vi "FTW-JSON-SerializeElement.vi"(0 "JSON Object":refnum<class "FTW-JSON.lvclass">, 5 "Key":string, 11 "error in":errorcluster) -> (4 "JSON Object":refnum<class "FTW-JSON.lvclass">, 6 "Element as JSON String":string, 10 "Found?":bool, 15 "error out":errorcluster)   [LabVIEW 2013, in "FTW-JSON.lvclass"]
uses:
  FTW-JSON.lvclass
  FTW-JSON.lvclass/FTW-JSON.ctl
panel:
  # "Inputs"
  # "Outputs"
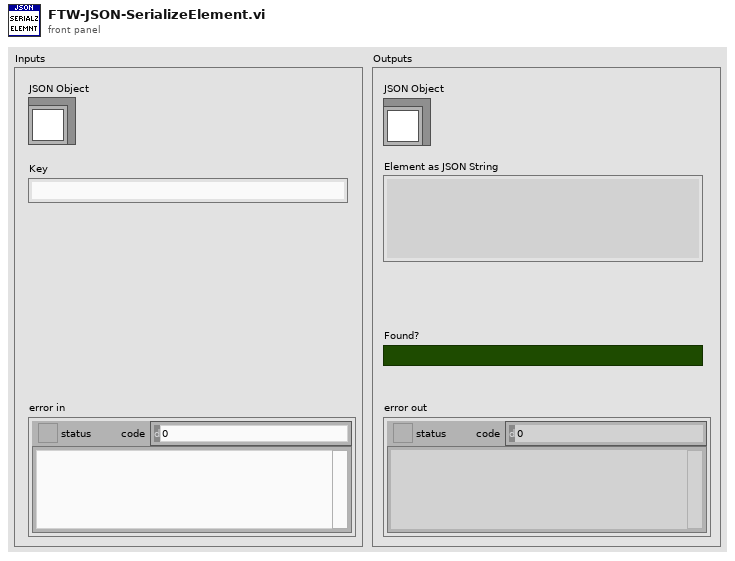
[diagram p1: front panel]
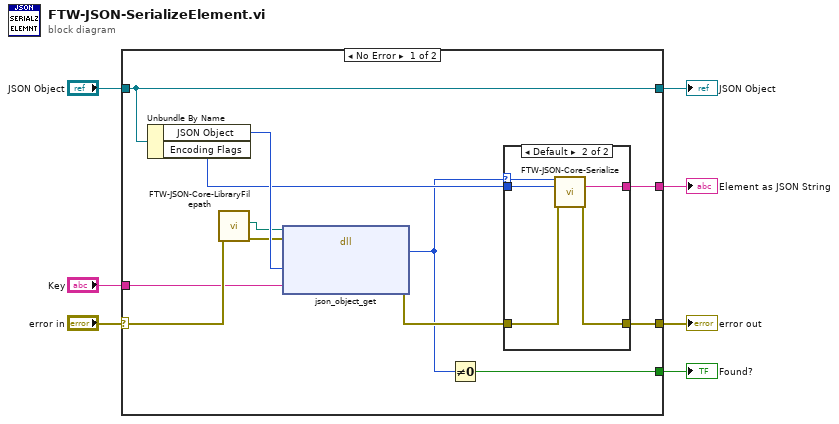
[diagram p0: block diagram]
diagram:
  n1 = case shown="No Error" "error in" {
    selector: "error in" -> [w19 w27]
    tunnel: [w10 w27] -> w7
    tunnel: [w13 w26] -> w5
    tunnel: "JSON Object" -> [w13 w26]
    tunnel: "Key" -> [w18 _]
    tunnel: [w17 _] -> w2
    tunnel: [w8 _] -> w1
    frame No Error {
      n2 = Unbundle By Name(w13) -> ("JSON Object"=w16:i64, "Encoding Flags"=w12:i64)
      n3 = call "FTW-JSON-Core-LibraryFilepath.vi"("error in"=w19) -> ("error out"=w15:errorcluster, "JSON Library Filepath"=w14:path)  [unwired: 9 in]
      n4 = dll-call lib="?" fn="json_object_get"(path in=w14, error in=w15, "JSON Object Pointer"=w16, "Element Key"=w18) -> (error out=w11:errorcluster, "JSON Element Pointer"=w9:i64)  [unwired: 3 in, 1 out]
      n5 = Not Equal To 0?(x=w9) -> (x != 0?=w17:bool)
      n6 = case shown="Default" w9 {
        selector: w9 -> [_ w22]
        tunnel: w12 -> [_ w25]
        tunnel: w11 -> [w20 w24]
        tunnel: [w20 w23] -> w10
        tunnel: [_ w21] -> w8
        frame 0 {
        }
        frame Default {
          n7 = call "FTW-JSON-Core-Serialize.vi"("JSON Object"=w22, "Encoding Flags"=w25, "error in"=w24) -> ("JSON String (UTF-8)"=w21:string, "error out"=w23:errorcluster)  [unwired: 10 in, 1 out]
        }
      }
    }
    frame Error {
    }
  }
  "error out" <- w7
  "JSON Object" <- w5
  "Found?" <- w2
  "Element as JSON String" <- w1
